vi "organize schedule.vi"(6 "periods per day":i32, 9 "Course ranking":i32[](array[numeric]), 11 "Student data":i32[][](array[numeric])) -> (3 "rearranged Student data":i32[][](array[numeric]))   [LabVIEW 2009]
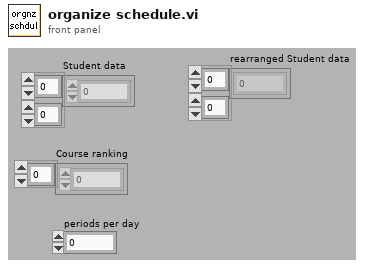
[diagram p1: front panel]
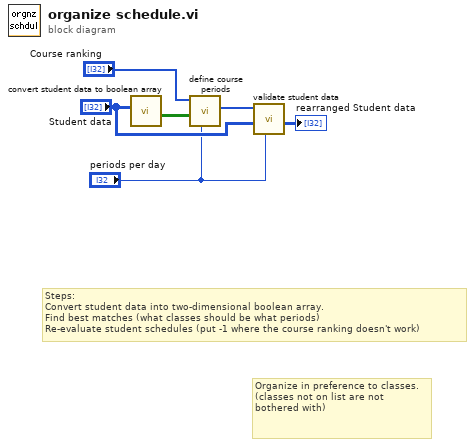
[diagram p0: block diagram]
diagram:
  # "Steps:\nConvert student data into two-dimensional boolean array.\nFind best matches (what classes should be what periods)\nRe-evaluate student schedules (put -1 where the course ranking doesn't work)"
  # "Organize in preference to classes.\n(classes not on list are not bothered with)"
  n1 = call "convert student data to boolean array.vi"("Student data"="Student data") -> ("expanded class data"=w5:bool[][])  [unwired: 10 in]
  n2 = call "define course periods.vi"("periods per day"="periods per day", "expanded class data"=w5, "Course ranking"="Course ranking") -> ("course periods"=w4:i32[])  [unwired: 8 in]
  n3 = call "validate student data.vi"("periods per day"="periods per day", "Student data"="Student data", "course periods"=w4) -> ("validated Student data"=→"rearranged Student data":i32[][])  [unwired: 8 in]
